vi "Configure Phase Noise Modulation.vi"(5 "Flat Phase Noise Power (-70 dBc/Hz)":dbl=-70.0, 6 "Stop Frequency (30000 Hz)":dbl=30000.0, 7 "Enable Phase Noise Impairment (F: Disable)":bool, 8 "error in (no error)":errorcluster, 9 "Start Frequency (1000 Hz)":dbl=1000.0, 10 "Modulation Format (0: Custom)":i32(ring) items=["Custom", "Vector Modulation"], 11 "VISA resource name":refnum<visa-resource-name>) -> (0 "error out":errorcluster, 3 "VISA resource name out":refnum<visa-resource-name>)   [LabVIEW 2012, in "Agilent PSG MXG Series.lvlib"]
doc: "Configure phase noise settings.\n\n<B>Notes:</B>\n(1) This VI is valid only in N5172B and N5182B that install <B>Option 660</B>."
uses:
  <instrlib>/Agilent PSG MXG Series/Agilent PSG MXG Series.lvlib
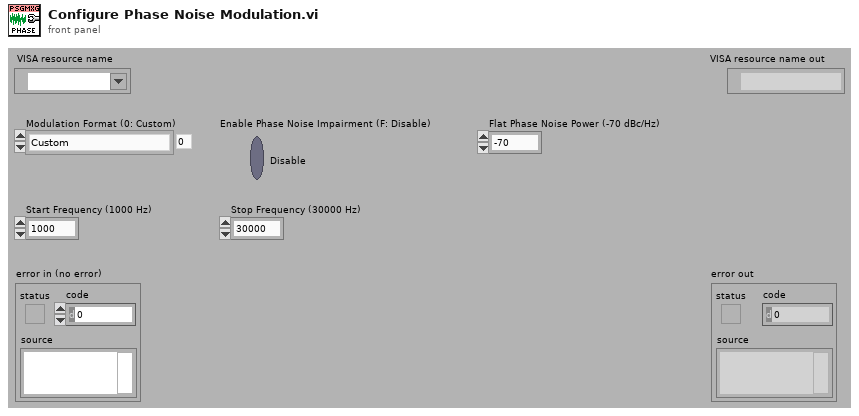
[diagram p1: front panel]
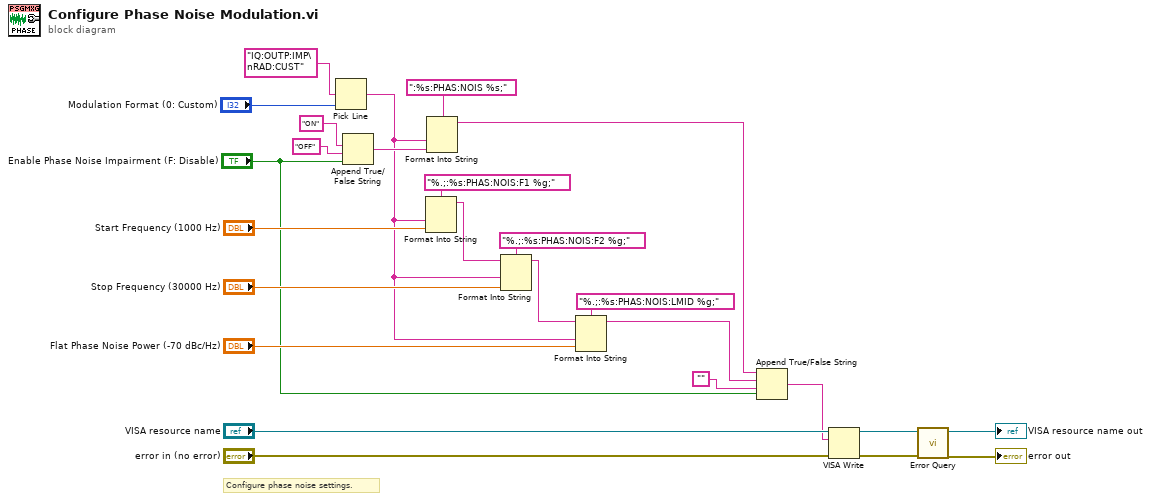
[diagram p0: block diagram]
diagram:
  # "Configure phase noise settings."
  n1 = Pick Line(multi-line string="IQ:OUTP:IMP\nRAD:CUST", line index="Modulation Format (0: Custom)") -> (output string=w7:string)  [unwired: 1 out]
  n2 = Append True/False String(1:"Enable Phase Noise Impairment (F: Disable)", 2:"OFF", 3:"ON") -> (0:w10:string)  [unwired: 1 out]
  n3 = Format Into String(format string="%.;:%s:PHAS:NOIS:F1 %g;", w7, "Start Frequency (1000 Hz)") -> (resulting string=w25:string)  [unwired: 2 in, 1 out]
  n4 = Format Into String(format string=":%s:PHAS:NOIS %s;", w7, w10) -> (resulting string=w5:string)  [unwired: 2 in, 1 out]
  n5 = Format Into String(format string="%.;:%s:PHAS:NOIS:F2 %g;", initial string=w25, w7, "Stop Frequency (30000 Hz)") -> (resulting string=w23:string)  [unwired: 1 in, 1 out]
  n6 = Format Into String(format string="%.;:%s:PHAS:NOIS:LMID %g;", initial string=w23, w7, "Flat Phase Noise Power (-70 dBc/Hz)") -> (resulting string=w3:string)  [unwired: 1 in, 1 out]
  n7 = Append True/False String(1:"Enable Phase Noise Impairment (F: Disable)", 2:"", 3:w3, 4:w5) -> (0:w1:string)
  n8 = VISA Write(VISA resource name="VISA resource name", write buffer=w1, error in (no error)="error in (no error)") -> (VISA resource name out=w19:refnum<visa-resource-name>, error out=w18:errorcluster)  [unwired: 1 out]
  n9 = call <instrlib>:"Error Query.vi"("error in (no error)"=w18, "VISA resource name"=w19) -> ("error out"=→"error out":errorcluster, "VISA resource name out"=→"VISA resource name out":refnum<visa-resource-name>)  [unwired: 8 out]
